vi "Create STAV.vi"(7 "baud rate (38400)":u32=38400, 8 "error in (no error)":errorcluster, 11 "STAV com port":refnum<visa-resource-name>) -> (0 "error out":errorcluster, 3 "STAV ref out":refnum<visa-resource-name>)   [LabVIEW 2021, in "STAV lib.lvlib"]
uses:
  STAV lib.lvlib
  <vilib>/Instr/_visa.llb/VISA Configure Serial Port (Instr).vi
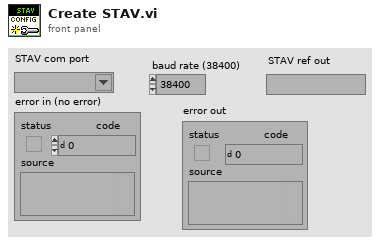
[diagram p1: front panel]
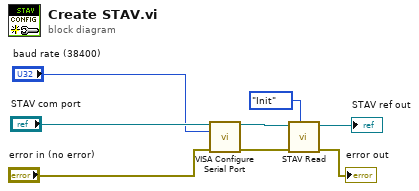
[diagram p0: block diagram]
diagram:
  n1 = call-poly "VISA Configure Serial Port"("VISA resource name"="STAV com port", "baud rate (9600)"="baud rate (38400)", "error in (no error)"="error in (no error)") -> ("VISA resource name out"=w3:refnum<visa-resource-name>, "error out"=w4:errorcluster)  [unwired: 11 in]
  n2 = call "STAV Read.vi"("Action (Read)"=enum16{"Read", "Init"}."Init" ("Action"), "error in (no error)"=w4, "STAV ref in"=w3) -> ("error out"=→"error out":errorcluster, "STAV ref out"=→"STAV ref out":refnum<visa-resource-name>)  [unwired: 5 in, 2 out]
